vi "Read Input and Output Channel Count.vi"(8 "error in":errorcluster, 11 "digital input and output mode in":refnum<class "Digital Input and Output Mode.lvclass">) -> (0 "error out":errorcluster, 1 "number output channels":i32, 2 "number input channels":i32, 3 "digital input and output mode out":refnum<class "Digital Input and Output Mode.lvclass">)   [LabVIEW 2020, in "Scan Engine Scripting.lvlib" / "Digital Input and Output Mode.lvclass"]
uses:
  Digital Input and Output Mode.lvclass
  Digital Input and Output Mode.lvclass/Digital Input and Output Mode.ctl
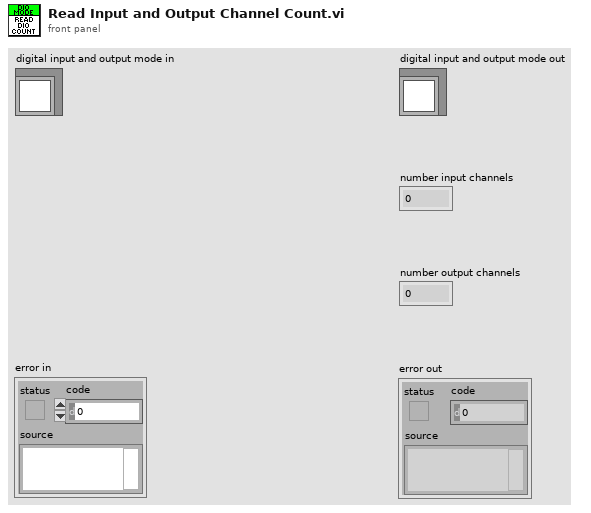
[diagram p1: front panel]
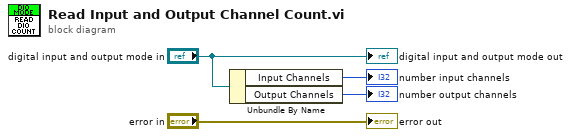
[diagram p0: block diagram]
diagram:
  n1 = Unbundle By Name("digital input and output mode in") -> ("Input Channels"=→"number input channels":i32, "Output Channels"=→"number output channels":i32)
  "error out" <- "error in"
  "digital input and output mode out" <- "digital input and output mode in"
